vi "_USB_Init.vi"(8 "Error In":errorcluster caption="错误输入") -> (0 "Error Out":errorcluster caption="错误输出", 3 "设备状态":bool)   [LabVIEW 2020, in "CH375.lvlib"]
uses:
  CH375.lvlib
  CH375DLL64.dll
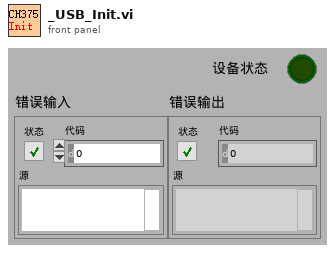
[diagram p1: front panel]
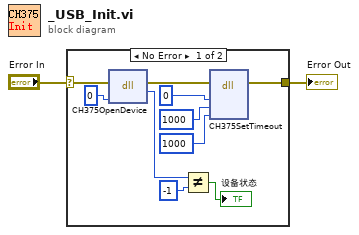
[diagram p0: block diagram]
diagram:
  n1 = case shown="No Error" "Error In" {
    selector: "Error In" -> [w6 w13]
    tunnel: [w4 w13] -> w2
    frame No Error {
      n2 = dll-call lib="D:/Project NJU/lib/CH375/CH375DLL64.dll" fn="CH375OpenDevice" ("打开CH376设备")(error in=w6, "index"=u32 0) -> (error out=w11:errorcluster, "handle"=w12:u16)  [unwired: 3 in, 1 out]
      n3 = Not Equal?(x=w12, y=i8 -1 ("x")) -> (x != y?=→"设备状态":bool)
      n4 = dll-call lib="D:/Project NJU/lib/CH375/CH375DLL64.dll" fn="CH375SetTimeout" ("设置超时")(error in=w11, "iIndex"=u32 0, "iWriteTimeout"=u32 1000, "iReadTimeout"=u32 1000) -> (error out=w4:errorcluster)  [unwired: 5 in, 2 out]
    }
    frame Error {
    }
  }
  "Error Out" <- w2
